vi "Initialize FPGA.vi"(8 "error in (no error)":errorcluster) -> (0 "error out":errorcluster, 3 "Generic FPGA Reference":T1)   [LabVIEW 2013, in "SGDV_Ctrl_v13_lib.lvlib"]
uses:
  SGDV_Ctrl_v13_lib.lvlib
  <vilib>/myRIO/Common/Instrument Driver Framework/Utilities/typedefs/Generic FPGA Reference.ctl
  <vilib>/rvi/interface/common/niFpgaWaitOnOcc.vi
  <vilib>/FPGAPlugInAG/myRIO-1900/niLvFpga_Open_myRIO-1900.vi
  <vilib>/rvi/interface/common/dynamic/niFpgaDynamicAddResources.vi
  <vilib>/Utility/error.llb/Error Cluster From Error Code.vi
  <vilib>/rvi/errors/niLvFpgaAdjustHostInterfaceError.vi
  <vilib>/myRIO/Common/Instrument Driver Framework/Utilities/vis/FPGA Ref Manager.vi
  <vilib>/FPGAPlugInAG/Dynamic/niLvFpga_Run_Dynamic.vi
  <vilib>/rvi/interface/nirviOpenFPGA/nirviOpenFPGA.xnode
  FPGA Bitfiles/DetalRobot_FPGATarget_FPGAMain(3Motor)_JiRD0S5fQ6s.lvbitx
  <vilib>/rvi/interface/nirviReadWriteControl/nirviReadWriteControl.xnode
  <vilib>/rvi/interface/nirviMethod/nirviMethod.xnode
  <vilib>/myRIO/Instrument Drivers/Utilities/Utilities.lvlib
  NiFpgaLv.dll
  <vilib>/rvi/interface/Simulation/niFpgaSimulationCallBeginRW.vi
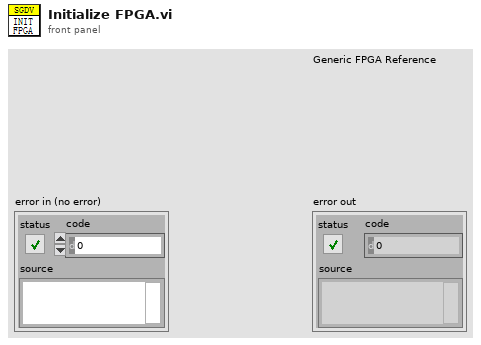
[diagram p1: front panel]
types:
  T1 = typedef "Generic FPGA Reference.ctl" = refnum<k20>
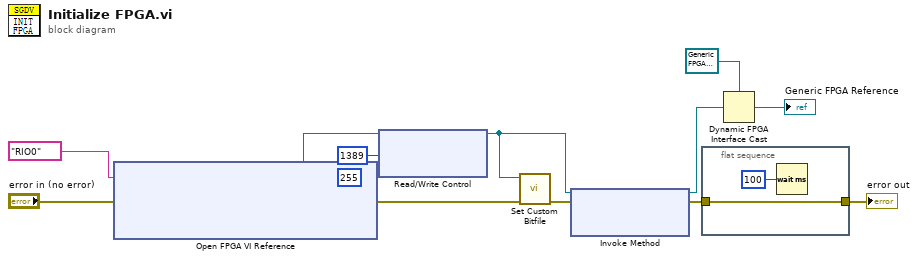
[diagram p0: block diagram]
diagram:
  n1 = xnode "Open FPGA VI Reference"("error in"="error in (no error)", "resource name"=tag "RIO0") -> ("FPGA VI Reference Out"=w8:refnum<k20>, "error out"=w12:errorcluster)
  n2 = xnode "Read/Write Control"("FPGA VI Reference In"=w8, "Recieved (ticks)"=u32 1389, "ABS Enc Channel"=u8 255) -> ("FPGA VI Reference Out"=w6:refnum<k20>)  [unwired: 1 in, 1 out]
  n3 = call <vilib>:"Set Custom Bitfile.vi"("error in (no error)"=w12, "Customized FPGA Reference in"=w6) -> ("error out"=w11:errorcluster)  [unwired: 8 in, 1 out]
  n4 = xnode "Invoke Method"("FPGA VI Reference In"=w6, "error in"=w11) -> ("FPGA VI Reference Out"=w2:refnum<k20>, "error out"=w5:errorcluster)  [unwired: 1 in]
  n5 = flat-sequence {
    tunnel: w5 -> [w14]
    tunnel: [w14] -> w4
    frame #0 {
      n6 = Wait (ms)(milliseconds to wait=u32 100) -> ()  [unwired: 1 out]
    }
  }
  n7 = Dynamic FPGA Interface Cast(Session In=T1 refnum ("Generic FPGA Reference"), Type=w2) -> (Session Out=→"Generic FPGA Reference":T1)
  "error out" <- w4
